vi "add set field(SubVI).vi"(10 "字符串":string) -> (0 "布尔 3":bool, 2 "连接的字符串":string)   [LabVIEW 2019, in "Add Seq.lvlib"]
uses:
  Add Seq.lvlib
  SubVI.lvlib
panel:
  in  "cancel":bool
  in  "ok":bool
  in  "Approach":i32(ring) items=["Linear", "NoOvershoot", "Oscillate"]
  in  "Mode":i32(ring) items=["Persistent", "Driven"]
  in  "Rate(Oe/min)":dbl=100.0 min=0.0 max=100.0
  in  "Field(Oe)":dbl min=-140000.0 max=140000.0
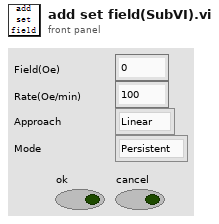
[diagram p1: front panel]
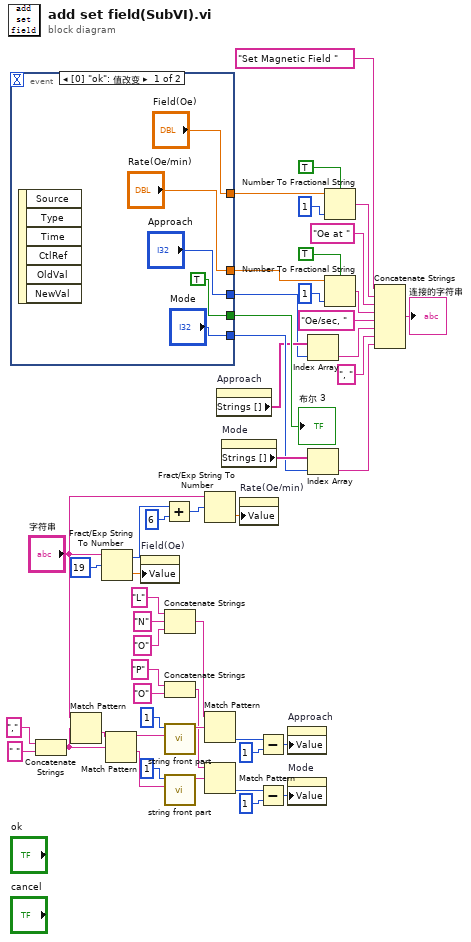
[diagram p0: block diagram]
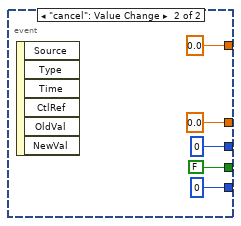
[diagram p2: hidden frame]
diagram:
  n1 = event shown="[0] \"ok\": 值改变" {
    selector: _ -> [_ _]
    dyn-events: _ -> [_ _]
    timeout: _ -> [_ _]
    tunnel: ["Rate(Oe/min)" 0.0 ("Rate输入")] -> w41
    tunnel: ["Field(Oe)" 0.0 ("Field")] -> w48
    tunnel: [TRUE FALSE] -> w50
    tunnel: ["Mode" 0 ("Mode输入")] -> w37
    tunnel: ["Approach" 0 ("Approach输入")] -> w34
    event "ok": Value Change {
      n2 = event-data() -> ()  [unwired: 1 in, 6 out]
    }
    event "cancel": Value Change {
      n3 = event-data() -> ()  [unwired: 1 in, 6 out]
    }
  }
  "布尔 3" <- w50
  n4 = Concatenate Strings("," ("字符串"), " " ("字符串")) -> (w6:string)
  n5 = Match Pattern(string="字符串", regular expression=w6) -> (after substring=w30:string)  [unwired: 1 in, 3 out]
  n6 = Fract/Exp String To Number(string="字符串", offset=19 ("偏移量")) -> (offset past number=w28:i32, number=w4:dbl)  [unwired: 2 in]
  n7 = Match Pattern(string=w30, regular expression=w6) -> (before substring=w11:string, after substring=w10:string)  [unwired: 1 in, 2 out]
  n8 = property on="Field(Oe)" class="DigNum (严格)"("Value"=w4) -> ()  [unwired: 2 in, 2 out]
  n9 = Add(x=w28, y=6) -> (x+y=w27:i32)
  n10 = Concatenate Strings("L" ("字符串"), "N" ("字符串"), "O" ("字符串")) -> (w20:string)
  n11 = Concatenate Strings("P" ("字符串"), "O" ("字符串")) -> (w13:string)
  n12 = call "string front part.vi"("字符串"=w11, "偏移量(0)"=1) -> ("result string"=w24:string)  [unwired: 9 in]
  n13 = call "string front part.vi"("字符串"=w10, "偏移量(0)"=1) -> ("result string"=w16:string)  [unwired: 9 in]
  n14 = Fract/Exp String To Number(string="字符串", offset=w27) -> (number=w3:dbl)  [unwired: 2 in, 1 out]
  n15 = Match Pattern(string=w20, regular expression=w24) -> (offset past match=w19:i32)  [unwired: 1 in, 3 out]
  n16 = Match Pattern(string=w13, regular expression=w16) -> (offset past match=w12:i32)  [unwired: 1 in, 3 out]
  n17 = property on="Approach" class="Ring (严格)"() -> ("Strings []"=w35:string[])  [unwired: 2 in, 2 out]
  n18 = property on="Mode" class="Ring (严格)"() -> ("Strings []"=w38:string[])  [unwired: 2 in, 2 out]
  n19 = property on="Rate(Oe/min)" class="DigNum (严格)"("Value"=w3) -> ()  [unwired: 2 in, 2 out]
  n20 = Subtract(x=w19, y=1) -> (x-y=w2:i32)
  n21 = Subtract(x=w12, y=1) -> (x-y=w1:i32)
  n22 = property on="Approach" class="Ring (严格)"("Value"=w2) -> ()  [unwired: 2 in, 2 out]
  n23 = property on="Mode" class="Ring (严格)"("Value"=w1) -> ()  [unwired: 2 in, 2 out]
  n24 = Index Array(array=w35, index=w34) -> (element=w32:string)
  n25 = Index Array(array=w38, index=w37) -> (element=w31:string)
  n26 = Number To Fractional String(use system decimal point (T)=TRUE ("使用系统小数点(T)"), number=w48, precision (6)=i16 1 ("精度(6)")) -> (F-format string=w46:string)  [unwired: 1 in]
  n27 = Number To Fractional String(use system decimal point (T)=TRUE ("使用系统小数点(T)"), number=w41, precision (6)=i16 1 ("精度(6)")) -> (F-format string=w40:string)  [unwired: 1 in]
  n28 = Concatenate Strings("Set Magnetic Field " ("字符串"), w46, "Oe at " ("字符串"), w40, "Oe/sec, " ("字符串"), w32, ", " ("字符串"), w31) -> (→"连接的字符串":string)
